vi "根据索引删除数组数据.vi"() -> ()   [LabVIEW 2017]
panel:
  out "元素":i32
  out "已删除的部分":dbl[][](array[numeric])
  out "已删除元素的数组子集":dbl[][](array[numeric])
  out "添加的数组 2":dbl[][](array[numeric])
  out "添加的数组":dbl[][](array[numeric])
  in  "数组":dbl[][](array[numeric])=[[1.0, 11.0, 21.0, 31.0, 41.0, 51.0, 61.0, 71.0, 81.0, 91.0], [2.0, 12.0, 22.0, 32.0, 42.0, 52.0, 62.0, 72.0, 82.0, 92.0], [3.0, 13.0, 23.0, 33.0, 43.0, 53.0, 63.0, 73.0, 83.0, 93.0], [4.0, 14.0, 24.0, 34.0, 44.0, 54.0, 64.0, 74.0, 84.0, 94.0], [5.0, 15.0, 25.0, 35.0, 45.0, 55.0, 65.0, 75.0, 85.0, 95.0], [6.0, 16.0, 26.0, 36.0, 46.0, 56.0, 66.0, 76.0, 86.0, 96.0], [7.0, 17.0, 27.0, 37.0, 47.0, 57.0, 67.0, 77.0, 87.0, 97.0], [8.0, 18.0, 28.0, 38.0, 48.0, 58.0, 68.0, 78.0, 88.0, 98.0], [9.0, 19.0, 29.0, 39.0, 49.0, 59.0, 69.0, 79.0, 89.0, 99.0]]
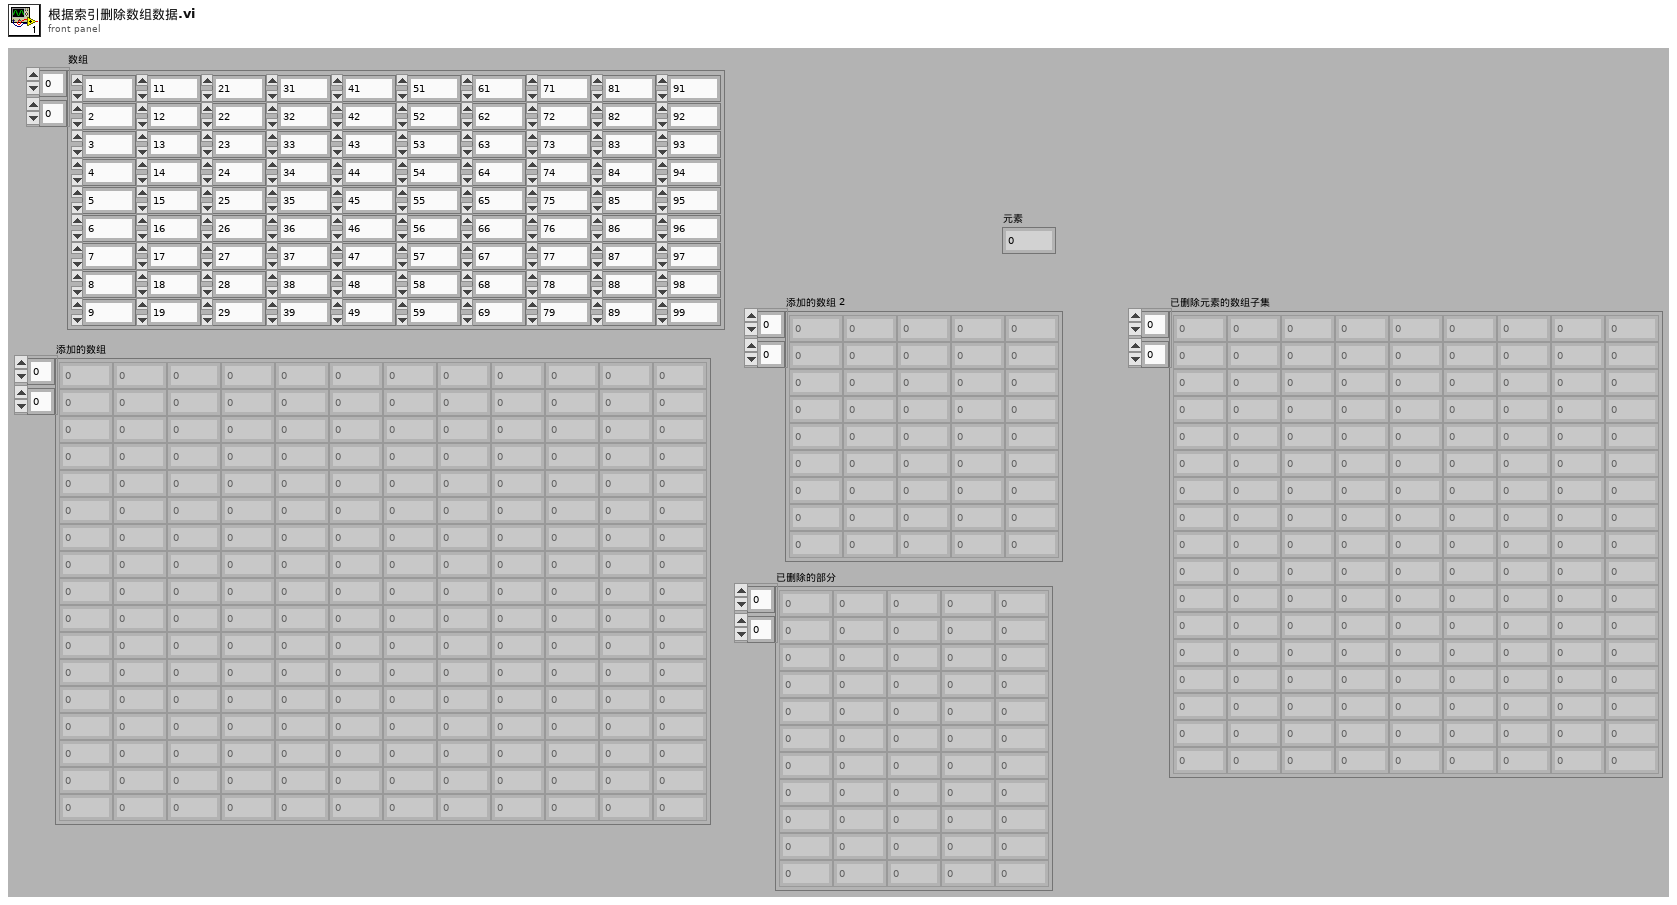
[diagram p1: front panel]
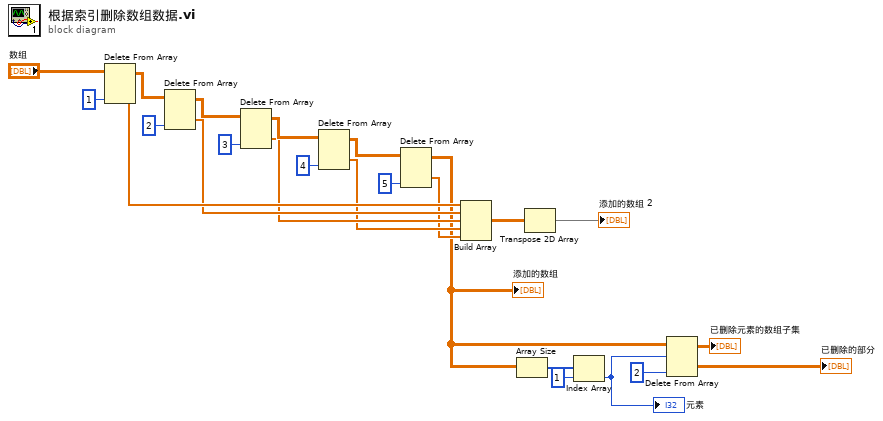
[diagram p0: block diagram]
diagram:
  n1 = Delete From Array(array="数组", index (col)=1 ("禁用的索引 (列)")) -> (deleted portion=w14:dbl[], array with subset deleted=w18:dbl[][])  [unwired: 2 in]
  n2 = Delete From Array(array=w18, index (col)=2 ("索引 (列)")) -> (deleted portion=w13:dbl[], array with subset deleted=w17:dbl[][])  [unwired: 2 in]
  n3 = Delete From Array(array=w17, index (col)=3 ("索引 (列)")) -> (deleted portion=w12:dbl[], array with subset deleted=w16:dbl[][])  [unwired: 2 in]
  n4 = Delete From Array(array=w16, index (col)=4 ("索引 (列)")) -> (deleted portion=w11:dbl[], array with subset deleted=w15:dbl[][])  [unwired: 2 in]
  n5 = Delete From Array(array=w15, index (col)=5 ("索引 (列)")) -> (deleted portion=w10:dbl[], array with subset deleted=w3:dbl[][])  [unwired: 2 in]
  "添加的数组" <- w3
  n6 = Build Array(w14, w13, w12, w11, w10) -> (w9:dbl[][])
  n7 = Array Size(array=w3) -> (size(s)=w6:i32[])
  n8 = Transpose 2D Array(2D array=w9) -> (transposed array=→"添加的数组 2":dbl[][])
  n9 = Index Array(array=w6, index=1 ("索引")) -> (element=w4:i32)
  "元素" <- w4
  n10 = Delete From Array(array=w3, length=w4, index (col)=2 ("索引 (行)")) -> (deleted portion=→"已删除的部分":dbl[][], array with subset deleted=→"已删除元素的数组子集":dbl[][])  [unwired: 1 in]
